vi "Custom Menu.vi"(8 "error in (no error)":errorcluster, 9 "\"New Components\" List":string[](array[string]), 10 "\"Active Components\" List":string[](array[string]), 11 "menu reference":refnum<k9>) -> (0 "error out":errorcluster, 2 "\"Active Component\" Item Tags Out":string[](array[string]), 3 "Menu out":refnum<k9>)   [LabVIEW 2023]
uses:
  Typedefs/Commands.ctl
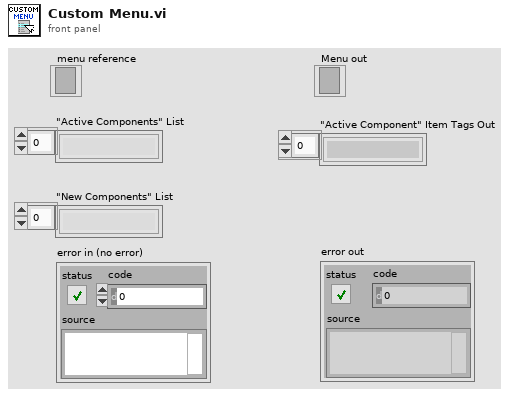
[diagram p1: front panel]
types:
  T1 = typedef "Commands.ctl" = enum16{"refresh", "listActiveComponents", "listComponents", "loadComponent", "unloadComponent", "swapComponent"}
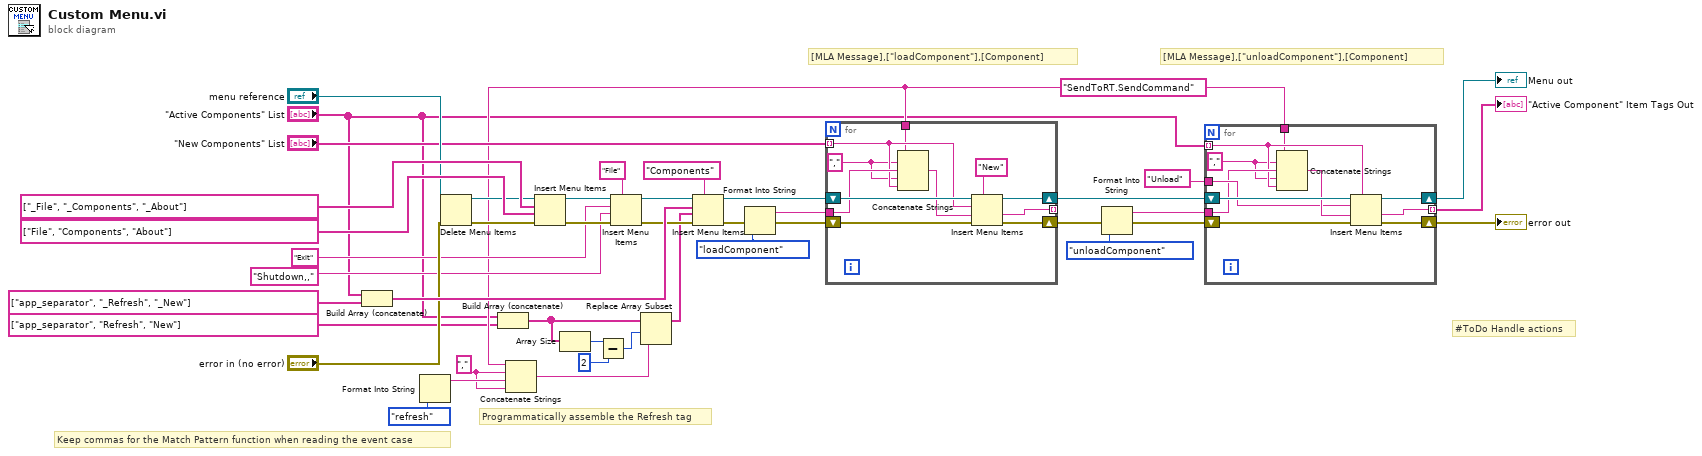
[diagram p0: block diagram]
diagram:
  w11 = ","
  w8 = "SendToRT.SendCommand"
  # "Programmatically assemble the Refresh tag"
  # "Keep commas for the Match Pattern function when reading the event case"
  # "[MLA Message],[\"loadComponent\"],[Component]"
  # "#ToDo Handle actions"
  # "[MLA Message],[\"unloadComponent\"],[Component]"
  n1 = Build Array (concatenate)("\"Active Components\" List", string[] ["app_separator", "_Refresh", "_New"] ("item tags")) -> (w37:string[])
  n2 = Format Into String(Commands."refresh") -> (resulting string=w12:string)  [unwired: 3 in, 1 out]
  n3 = Delete Menu Items(6:"error in (no error)", 9:"menu reference") -> (0:w32:errorcluster, 3:w29:refnum<k9>)  [unwired: 2 in]
  n4 = Build Array (concatenate)("\"Active Components\" List", string[] ["app_separator", "Refresh", "New"] ("item tags")) -> (w4:string[])
  n5 = Concatenate Strings(w8, w11, w12, w11) -> (w10:string)
  n6 = Insert Menu Items(6:w32, 7:string[] ["File", "Components", "About"] ("item tags"), 8:string[] ["_File", "_Components", "_About"] ("item tags"), 9:w29) -> (0:w42:errorcluster, 3:w27:refnum<k9>)  [unwired: 2 in, 1 out]
  n7 = Array Size(array=w4) -> (size(s)=w3:i32)
  n8 = Subtract(x=w3, y=2) -> (x-y=w2:i32)
  n9 = Insert Menu Items(5:"File" ("menu tag"), 6:w42, 7:"Shutdown,,", 8:"Exit", 9:w27) -> (0:w28:errorcluster, 3:w26:refnum<k9>)  [unwired: 1 in, 1 out]
  n10 = Replace Array Subset(array=w4, new element=w10, index=w2) -> (w9:string[])
  n11 = Insert Menu Items(5:"Components" ("menu tag"), 6:w28, 7:w9, 8:w37, 9:w26) -> (0:w21:errorcluster, 3:w40:refnum<k9>)  [unwired: 1 in, 1 out]
  n12 = Format Into String(error in=w21, Commands."loadComponent") -> (resulting string=w17:string, error out=w20:errorcluster)  [unwired: 2 in]
  n13 = for {
    shift-right: [w52] -> w18
    shift-left: w40 -> [w53]
    shift-right: [w44] -> w5
    shift-left: w20 -> [w54]
    tunnel: "\"New Components\" List" -> [w48] mode=indexing
    tunnel: [w51] -> _ mode=indexing
    tunnel: w17 -> [w49]
    tunnel: w8 -> [w46]
    w45 = "," ("string")
    n14 = Concatenate Strings(w46, w45, w49, w45, w48) -> (w50:string)
    n15 = Insert Menu Items(5:"New", 6:w54, 7:w50, 8:w48, 9:w53) -> (0:w44:errorcluster, 1:w51:string, 3:w52:refnum<k9>)  [unwired: 1 in]
  }
  n16 = Format Into String(error in=w5, Commands."unloadComponent") -> (resulting string=w22:string, error out=w24:errorcluster)  [unwired: 2 in]
  n17 = for {
    shift-right: [w63] -> w39
    shift-left: w18 -> [w64]
    shift-right: [w55] -> w38
    shift-left: w24 -> [w65]
    tunnel: "Unload" -> [w60]
    tunnel: [w62] -> w35 mode=indexing
    tunnel: w22 -> [w59]
    tunnel: "\"Active Components\" List" -> [w58] mode=indexing
    tunnel: w8 -> [w57]
    w56 = "," ("string")
    n18 = Concatenate Strings(w57, w56, w59, w56, w58) -> (w61:string)
    n19 = Insert Menu Items(5:w58, 6:w65, 7:w61, 8:w60, 9:w64) -> (0:w55:errorcluster, 1:w62:string, 3:w63:refnum<k9>)  [unwired: 1 in]
  }
  "Menu out" <- w39
  "error out" <- w38
  "\"Active Component\" Item Tags Out" <- w35
